vi "Initialize.vi"(8 "error in":errorcluster, 11 "Plugin in":refnum<class "Sift TDMS Uploader.lvclass">) -> (0 "error out":errorcluster, 3 "Plugin out":refnum<class "Sift TDMS Uploader.lvclass">)   [LabVIEW 2024, in "Sift TDMS Uploader.lvlib" / "Sift TDMS Uploader.lvclass"]
uses:
  Sift TDMS Uploader.lvclass
  C:/Program Files/National Instruments/LabVIEW 2024/vi.lib/FlexLogger/SDK/PluginSDK.lvlibp/PEFClasses/SDK/Plugin/Plugin.lvclass
  C:/Program Files/National Instruments/LabVIEW 2024/vi.lib/FlexLogger/SDK/PluginSDK.lvlibp/PEFClasses/SDK/Processing Element/Processing Element.lvclass
  <vilib>/FlexLogger/SDK/PluginSDK.lvlibp/PEFClasses/SDK/Processing Element/Timing Parameters.ctl
  <vilib>/FlexLogger/SDK/PluginSDK.lvlibp/PEFClasses/SDK/Processing Element/Timing Method.ctl
  <vilib>/FlexLogger/SDK/PluginSDK.lvlibp/PEFClasses/SDK/Plugin/ParameterAccess/Write String.vi
  <vilib>/FlexLogger/SDK/PluginSDK.lvlibp/PEFClasses/SDK/Processing Element/Read System Interface.vi
  <vilib>/FlexLogger/SDK/PluginSDK.lvlibp/PEFClasses/SDK/Processing Element/Read Alias.vi
  Globals.vi
  <vilib>/FlexLogger/SDK/PluginSDK.lvlibp/PEFClasses/SDK/Plugin/Plugin.lvclass
  <vilib>/FlexLogger/SDK/PluginSDK.lvlibp/PEFClasses/SDK/System Interface/System Interface.lvclass
  <vilib>/FlexLogger/SDK/PluginSDK.lvlibp/PEFClasses/SDK/Processing Element/Processing Element.lvclass
  C:/Users/Alex luCK/Documents/Projects/sift-labview/plugins/flexlogger/Sift TDMS Uploader/Sift TDMS Uploader.lvclass
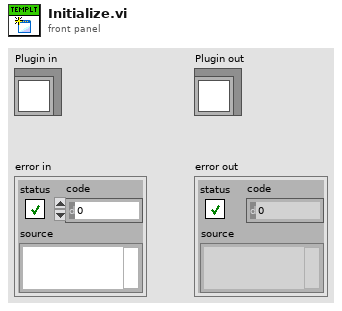
[diagram p1: front panel]
types:
  T1 = typedef "PluginSDK.lvlibp/Processing Element.lvclass/Timing Parameters.ctl" = cluster{"Timing Method":T2, "Timing Period (ms)":i32}
  T2 = typedef "PluginSDK.lvlibp/Processing Element.lvclass/Timing Method.ctl" = enum16{"Periodic", "Immediate", "On Data Ready", "Triggered"}
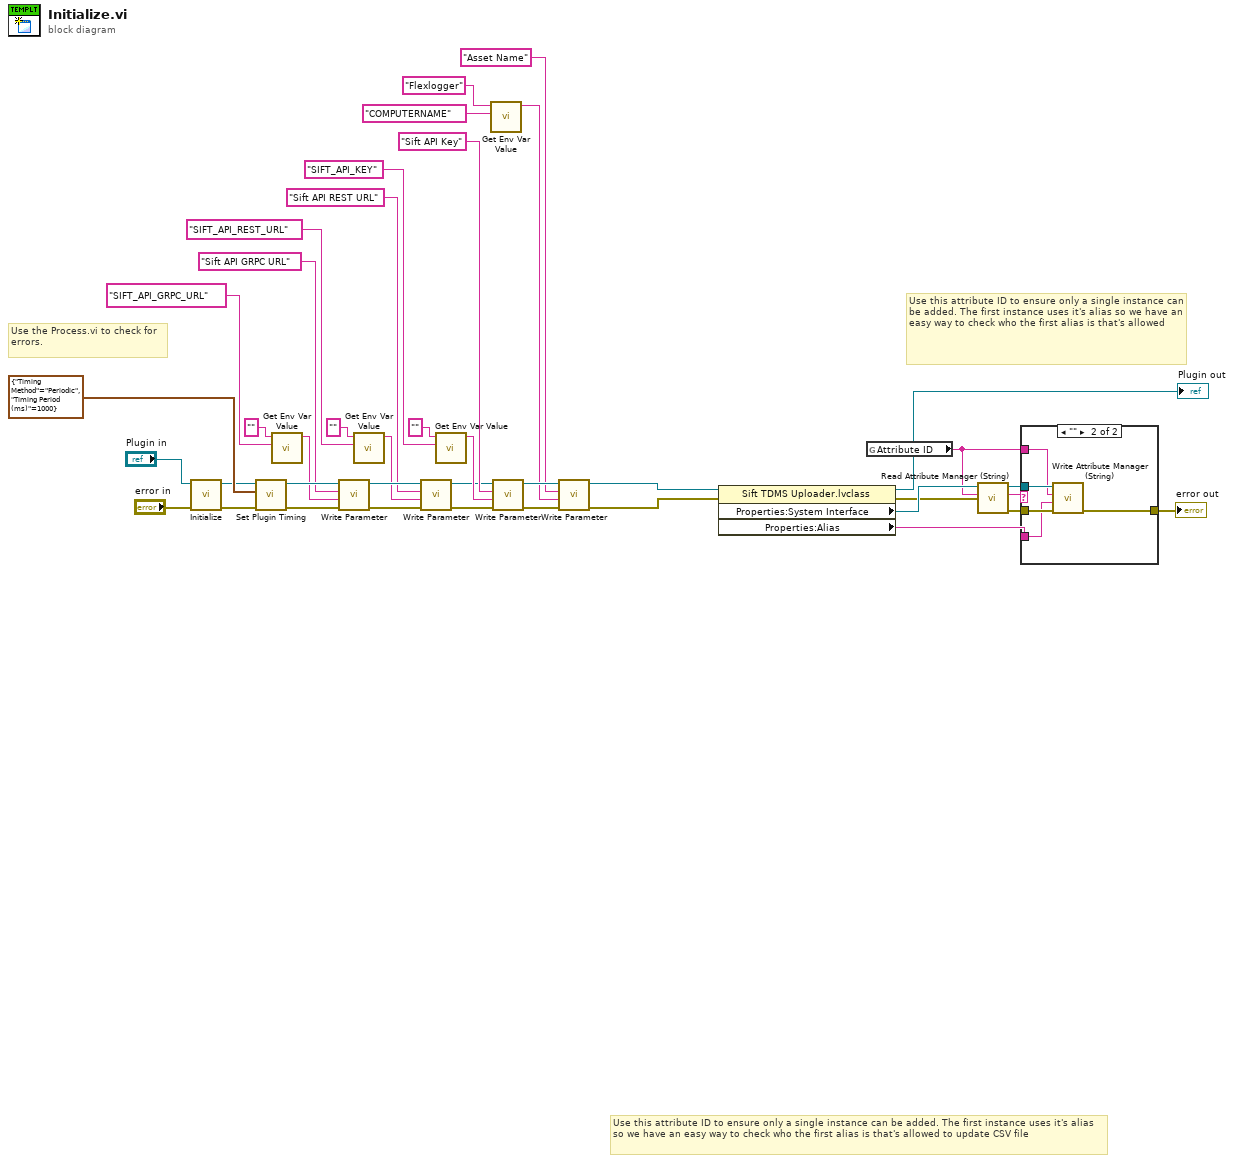
[diagram p0: block diagram]
diagram:
  # "Use this attribute ID to ensure only a single instance can be added. The first instance uses it's alias so we have an easy way to check who the first alias is that's allowed to update CSV file"
  # "Use the Process.vi to check for errors."
  # "Use this attribute ID to ensure only a single instance can be added. The first instance uses it's alias so we have an easy way to check who the first alias is that's allowed"
  n1 = call-parent "Initialize.vi"("error in (no error)"="error in", "Plugin in"="Plugin in") -> ("error out"=w37:errorcluster, "Plugin out"=w36:refnum<class "Sift TDMS Uploader.lvclass">)  [unwired: 8 in]
  n2 = call <vilib>:"Set Plugin Timing.vi"("error in (no error)"=w37, "Timing Parameters"=T1 {"Timing Method"=enum."Periodic", "Timing Period (ms)"=1000}, "Plugin in"=w36) -> ("error out"=w34:errorcluster, "Plugin out"=w35:refnum<class "Sift TDMS Uploader.lvclass">)  [unwired: 7 in]
  n3 = call "Get Env Var Value.vi"("env var name"="SIFT_API_GRPC_URL", "default value"="") -> ("result"=w31:string)  [unwired: 9 in]
  n4 = call-poly <vilib>:"Write Parameter.vi"("error in (no error)"=w34, "Value"=w31, "Name"="Sift API GRPC URL", "Plugin in"=w35) -> ("error out"=w17:errorcluster, "Plugin out"=w19:refnum<class "Sift TDMS Uploader.lvclass">)  [unwired: 6 in]
  n5 = call "Get Env Var Value.vi"("env var name"="SIFT_API_REST_URL", "default value"="") -> ("result"=w13:string)  [unwired: 9 in]
  n6 = call-poly <vilib>:"Write Parameter.vi"("error in (no error)"=w17, "Value"=w13, "Name"="Sift API REST URL", "Plugin in"=w19) -> ("error out"=w16:errorcluster, "Plugin out"=w18:refnum<class "Sift TDMS Uploader.lvclass">)  [unwired: 6 in]
  n7 = call "Get Env Var Value.vi"("env var name"="SIFT_API_KEY", "default value"="") -> ("result"=w26:string)  [unwired: 9 in]
  n8 = call "Get Env Var Value.vi"("env var name"="COMPUTERNAME", "default value"="Flexlogger") -> ("result"=w9:string)  [unwired: 9 in]
  n9 = call-poly <vilib>:"Write Parameter.vi"("error in (no error)"=w16, "Value"=w26, "Name"="Sift API Key", "Plugin in"=w18) -> ("error out"=w29:errorcluster, "Plugin out"=w30:refnum<class "Sift TDMS Uploader.lvclass">)  [unwired: 6 in]
  n10 = call-poly <vilib>:"Write Parameter.vi"("error in (no error)"=w29, "Value"=w9, "Name"="Asset Name", "Plugin in"=w30) -> ("error out"=w2:errorcluster, "Plugin out"=w1:refnum<class "Sift TDMS Uploader.lvclass">)  [unwired: 6 in]
  n11 = property class="Sift TDMS Uploader.lvclass"(reference=w1, error in=w2) -> (reference out=→"Plugin out":refnum<class "Sift TDMS Uploader.lvclass">, error out=w23:errorcluster, "Properties:System Interface"=w24:refnum<class "System Interface.lvclass">, "Properties:Alias"=w6:string)
  n12 = global read "Globals.vi" "Attribute ID"() -> (w3:string)
  n13 = call-dynamic "Read Attribute Manager (String).vi"("error in (no error)"=w23, "Attribute ID"=w3, "System Interface in"=w24) -> ("error out"=w7:errorcluster, "Attrib Val"=w4:string, "System Interface out"=w5:refnum<class "System Interface.lvclass">)  [unwired: 5 in, 1 out]
  n14 = case shown="\"\"" w4 {
    tunnel: w5 -> [_ w46]
    tunnel: w7 -> [w41 w45]
    tunnel: w6 -> [_ w43]
    tunnel: w3 -> [_ w44]
    tunnel: [w41 w42] -> w8
    frame Default {
      # "An instance already exists. Let Process.vi return error"
    }
    frame "" {
      n15 = call-dynamic "Write Attribute Manager (String).vi"("error in (no error)"=w45, "Attribute Value"=w43, "Attribute ID"=w44, "System Interface in"=w46) -> ("error out"=w42:errorcluster)  [unwired: 5 in, 2 out]
    }
  }
  "error out" <- w8
